vi "Log Events.vi"(8 "error in":errorcluster, 9 "session id":u64, 10 "log directory path":path, 11 "event records":string[](array[string])) -> (0 "error out":errorcluster)   [LabVIEW 2021, in "Game of Life.lvlib"]
doc: "Logs the recorded events to a CSV file."
uses:
  Game of Life.lvlib
  <vilib>/Utility/file.llb/Write Delimited Spreadsheet (string).vi
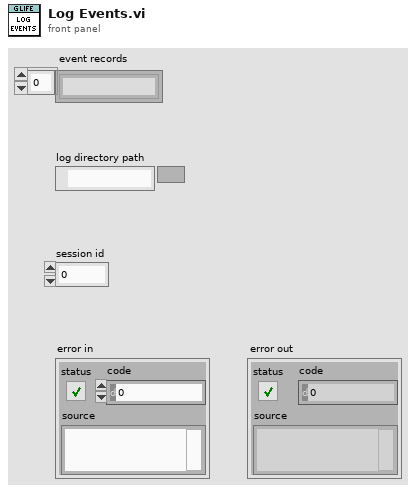
[diagram p1: front panel]
types:
  T1 = enum16{"open", "replace", "create", "open or create", "replace or create", "replace or create with confirmation"}
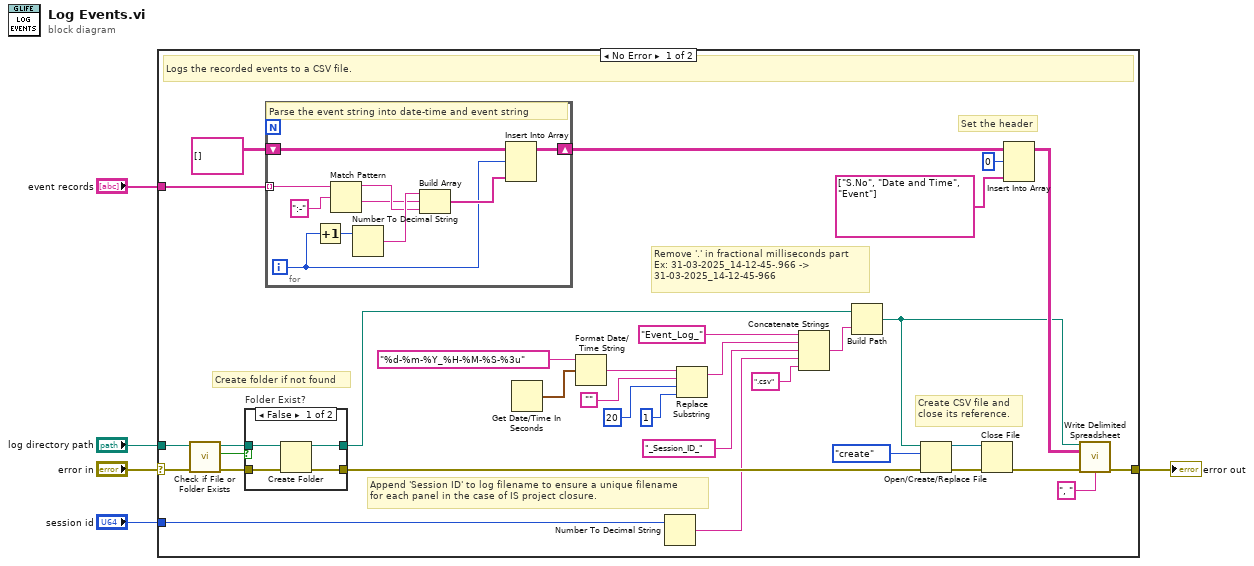
[diagram p0: block diagram]
diagram:
  n1 = case shown="No Error" "error in" {
    selector: "error in" -> [w36 w55]
    tunnel: [w32 w55] -> w5
    tunnel: "log directory path" -> [w29 _]
    tunnel: "event records" -> [w9 _]
    tunnel: "session id" -> [w7 _]
    frame No Error {
      # "Remove '.' in fractional milliseconds part\nEx: 31-03-2025_14-12-45-.966 ->\n31-03-2025_14-12-45-966"
      # "Append 'Session ID' to log filename to ensure a unique filename\nfor each panel in the case of IS project closure."
      # "Create CSV file and \nclose its reference."
      # "Create folder if not found"
      # "Set the header"
      # "Logs the recorded events to a CSV file."
      n2 = call <vilib>:"Check if File or Folder Exists.vi"("error in (no error)"=w36, "path"=w29) -> ("error out"=w35:errorcluster, "file or folder exists?"=w30:bool, "dup path"=w31:path)  [unwired: 7 in]
      n3 = case "Folder Exist?" shown="False" w30 {
        tunnel: w35 -> [w42 w44]
        tunnel: [w41 w44] -> w34
        tunnel: w31 -> [w40 w43]
        tunnel: [w39 w43] -> w6
        frame False {
          n4 = Create Folder(path (use dialog)=w40, error in=w42) -> (created path=w39:path, error out=w41:errorcluster)  [unwired: 1 in, 1 out]
        }
        frame True {
        }
      }
      n5 = for {
        tunnel: w9 -> [w47] mode=indexing
        shift-right: [w52] -> w10
        shift-left: string[][] [] ("Item Names") -> [w53]
        i -> [w45]
        # "Parse the event string into date-time and event string"
        n6 = Increment(x=w45) -> (x+1=w54:i32)
        n7 = Match Pattern(string=w47, regular expression=":-") -> (before substring=w49:string, after substring=w48:string)  [unwired: 1 in, 2 out]
        n8 = Number To Decimal String(number=w54) -> (decimal integer string=w50:string)  [unwired: 1 in]
        n9 = Build Array(w50, w48, w49) -> (w51:string[])
        n10 = Insert Into Array(array=w53, index (row)=w45, new element=w51) -> (w52:string[][])  [unwired: 1 in]
      }
      n11 = Get Date/Time In Seconds() -> (seconds since 1Jan1904=w21:timestamp)
      n12 = Format Date/Time String(time format string (%c)="%d-%m-%Y_%H-%M-%S-%3u", seconds (now)=w21) -> (date/time string=w26:string)  [unwired: 1 in]
      n13 = Number To Decimal String(number=w7) -> (decimal integer string=w19:string)  [unwired: 1 in]
      n14 = Replace Substring(2:1 ("length (len. of substring)"), 3:20 ("offset (0)"), 4:"" ("substring (\"\")"), 5:w26) -> (1:w20:string)  [unwired: 1 out]
      n15 = Concatenate Strings("Event_Log_" ("string"), w20, "_Session_ID_" ("string"), w19, ".csv" ("string")) -> (w15:string)
      n16 = Build Path(base path=w6, name or relative path=w15) -> (appended path=w12:path)
      n17 = Open/Create/Replace File(file path (use dialog)=w12, error in=w34, operation (0:open)=T1."create") -> (refnum out=w37:refnum<file>, error out=w38:errorcluster)  [unwired: 3 in, 1 out]
      n18 = Close File(refnum=w37, error in=w38) -> (error out=w28:errorcluster)  [unwired: 1 out]
      n19 = Insert Into Array(array=w10, index (row)=0, new element=string[] ["S.No", "Date and Time", "Event"] ("new element/subarray")) -> (w33:string[][])  [unwired: 1 in]
      n20 = call-poly <vilib>:"Write Delimited Spreadsheet.vi"("file path (dialog if empty)"=w12, "2D data"=w33, "error in (no error)"=w28, "delimiter (\\t)"=", " ("delimiter (\\t)")) -> ("error out"=w32:errorcluster)  [unwired: 10 in, 1 out]
    }
    frame Error {
    }
  }
  "error out" <- w5
